vi "SubVI_LightCommand.vi"(9 "命令值":u8, 10 "亮度":u8, 11 "通道":u8=1 min=1 max=4) -> (3 "concatenated string":string)   [LabVIEW 2015]
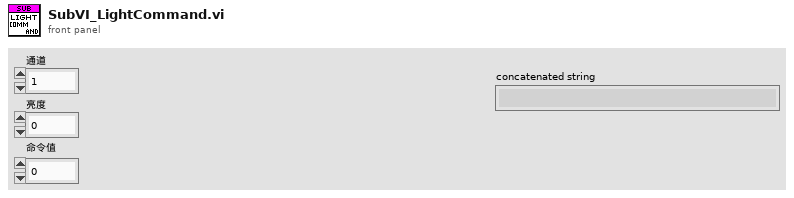
[diagram p1: front panel]
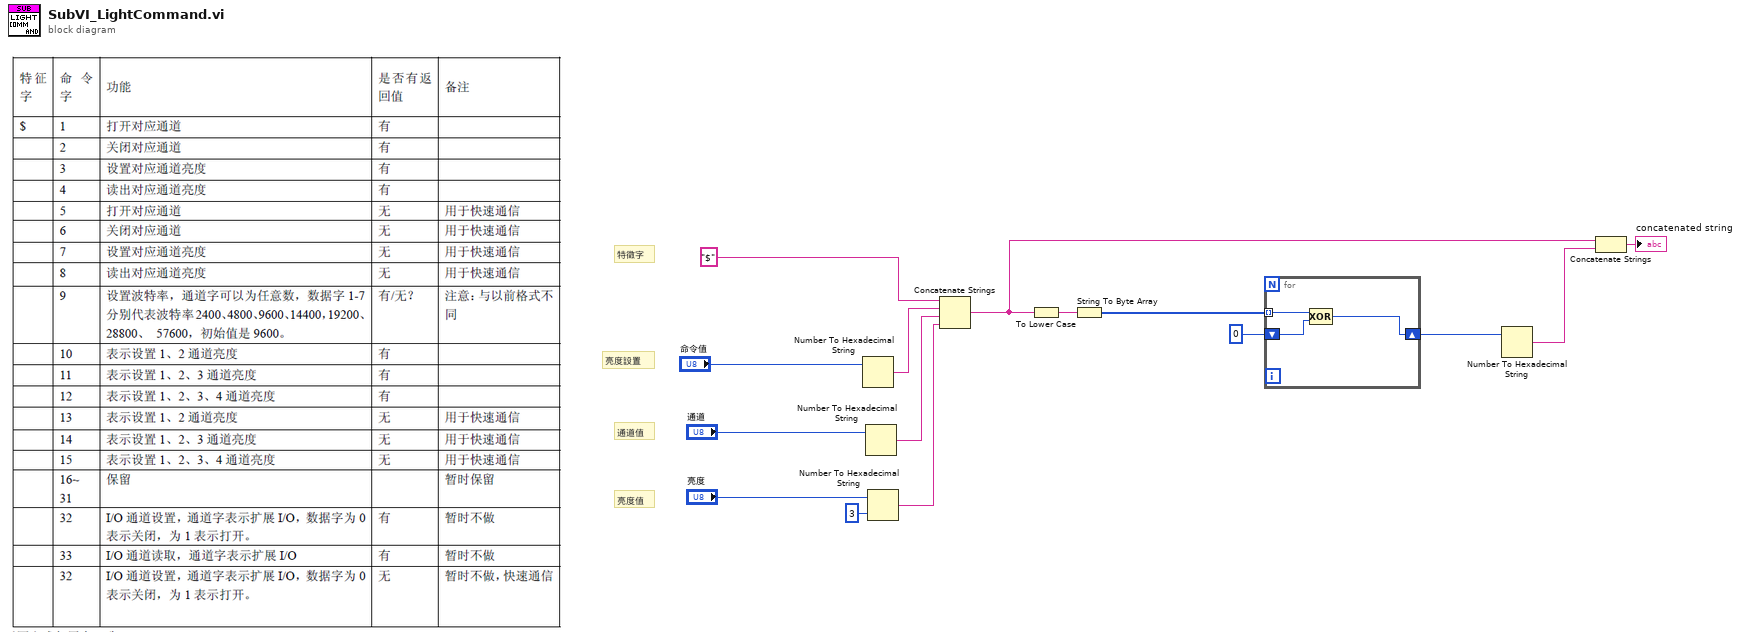
[diagram p0: block diagram]
diagram:
  # "亮度值"
  # "通道值"
  # "亮度設置"
  # "特徵字"
  n1 = Number To Hexadecimal String(2:"命令值") -> (0:w14:string)  [unwired: 1 in]
  n2 = Number To Hexadecimal String(2:"通道") -> (0:w13:string)  [unwired: 1 in]
  n3 = Number To Hexadecimal String(1:i16 3 ("width (-)"), 2:"亮度") -> (0:w12:string)
  n4 = Concatenate Strings("$" ("string"), w14, w13, w12) -> (w6:string)
  n5 = To Lower Case(string=w6) -> (all lower case string=w10:string)
  n6 = String To Byte Array(string=w10) -> (unsigned byte array=w9:u8[])
  n7 = for {
    tunnel: w9 -> [w17] mode=indexing
    shift-right: [w18] -> w7
    shift-left: u8 0 -> [w16]
    n8 = Compound Arithmetic op=XOR(w17, w16) -> (w18:u8)
  }
  n9 = Number To Hexadecimal String(2:w7) -> (0:w5:string)  [unwired: 1 in]
  n10 = Concatenate Strings(w6, w5) -> (→"concatenated string":string)
